vi "BRig_RT__Case_Exp__State_initBlock__v10.vi"(0 "input_dataCurrent":u16[](array[numeric]), 3 "input_dataExp":u16[](array[numeric]), 4 "input_dataBlock":u16[][](array[numeric]), 5 "input_dataTrial":u16[][](array[numeric])) -> (6 "output_iSpout":u16, 7 "output_speaker_amp_R":u16, 8 "output_iBlock":u16, 9 "output_speaker_freq_R":u8, 10 "output_BUR_target":u16, 11 "output_speaker_amp_L":u16, 12 "output_TpB_target":u16, 13 "output_speaker_freq_L":u8, 14 "output_dataCurrent":u16[](array[numeric]), 18 "output_dataBlock":u16[][](array[numeric]), 19 "output_dataTrial":u16[][](array[numeric]))   [LabVIEW 2014]
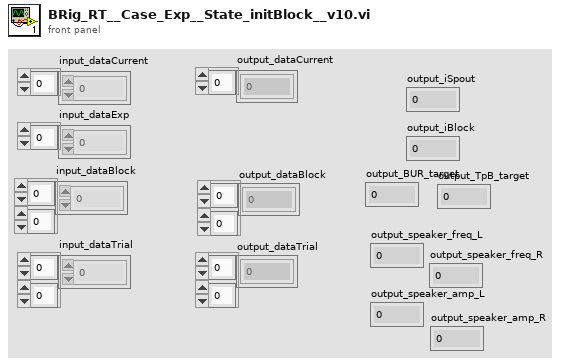
[diagram p1: front panel]
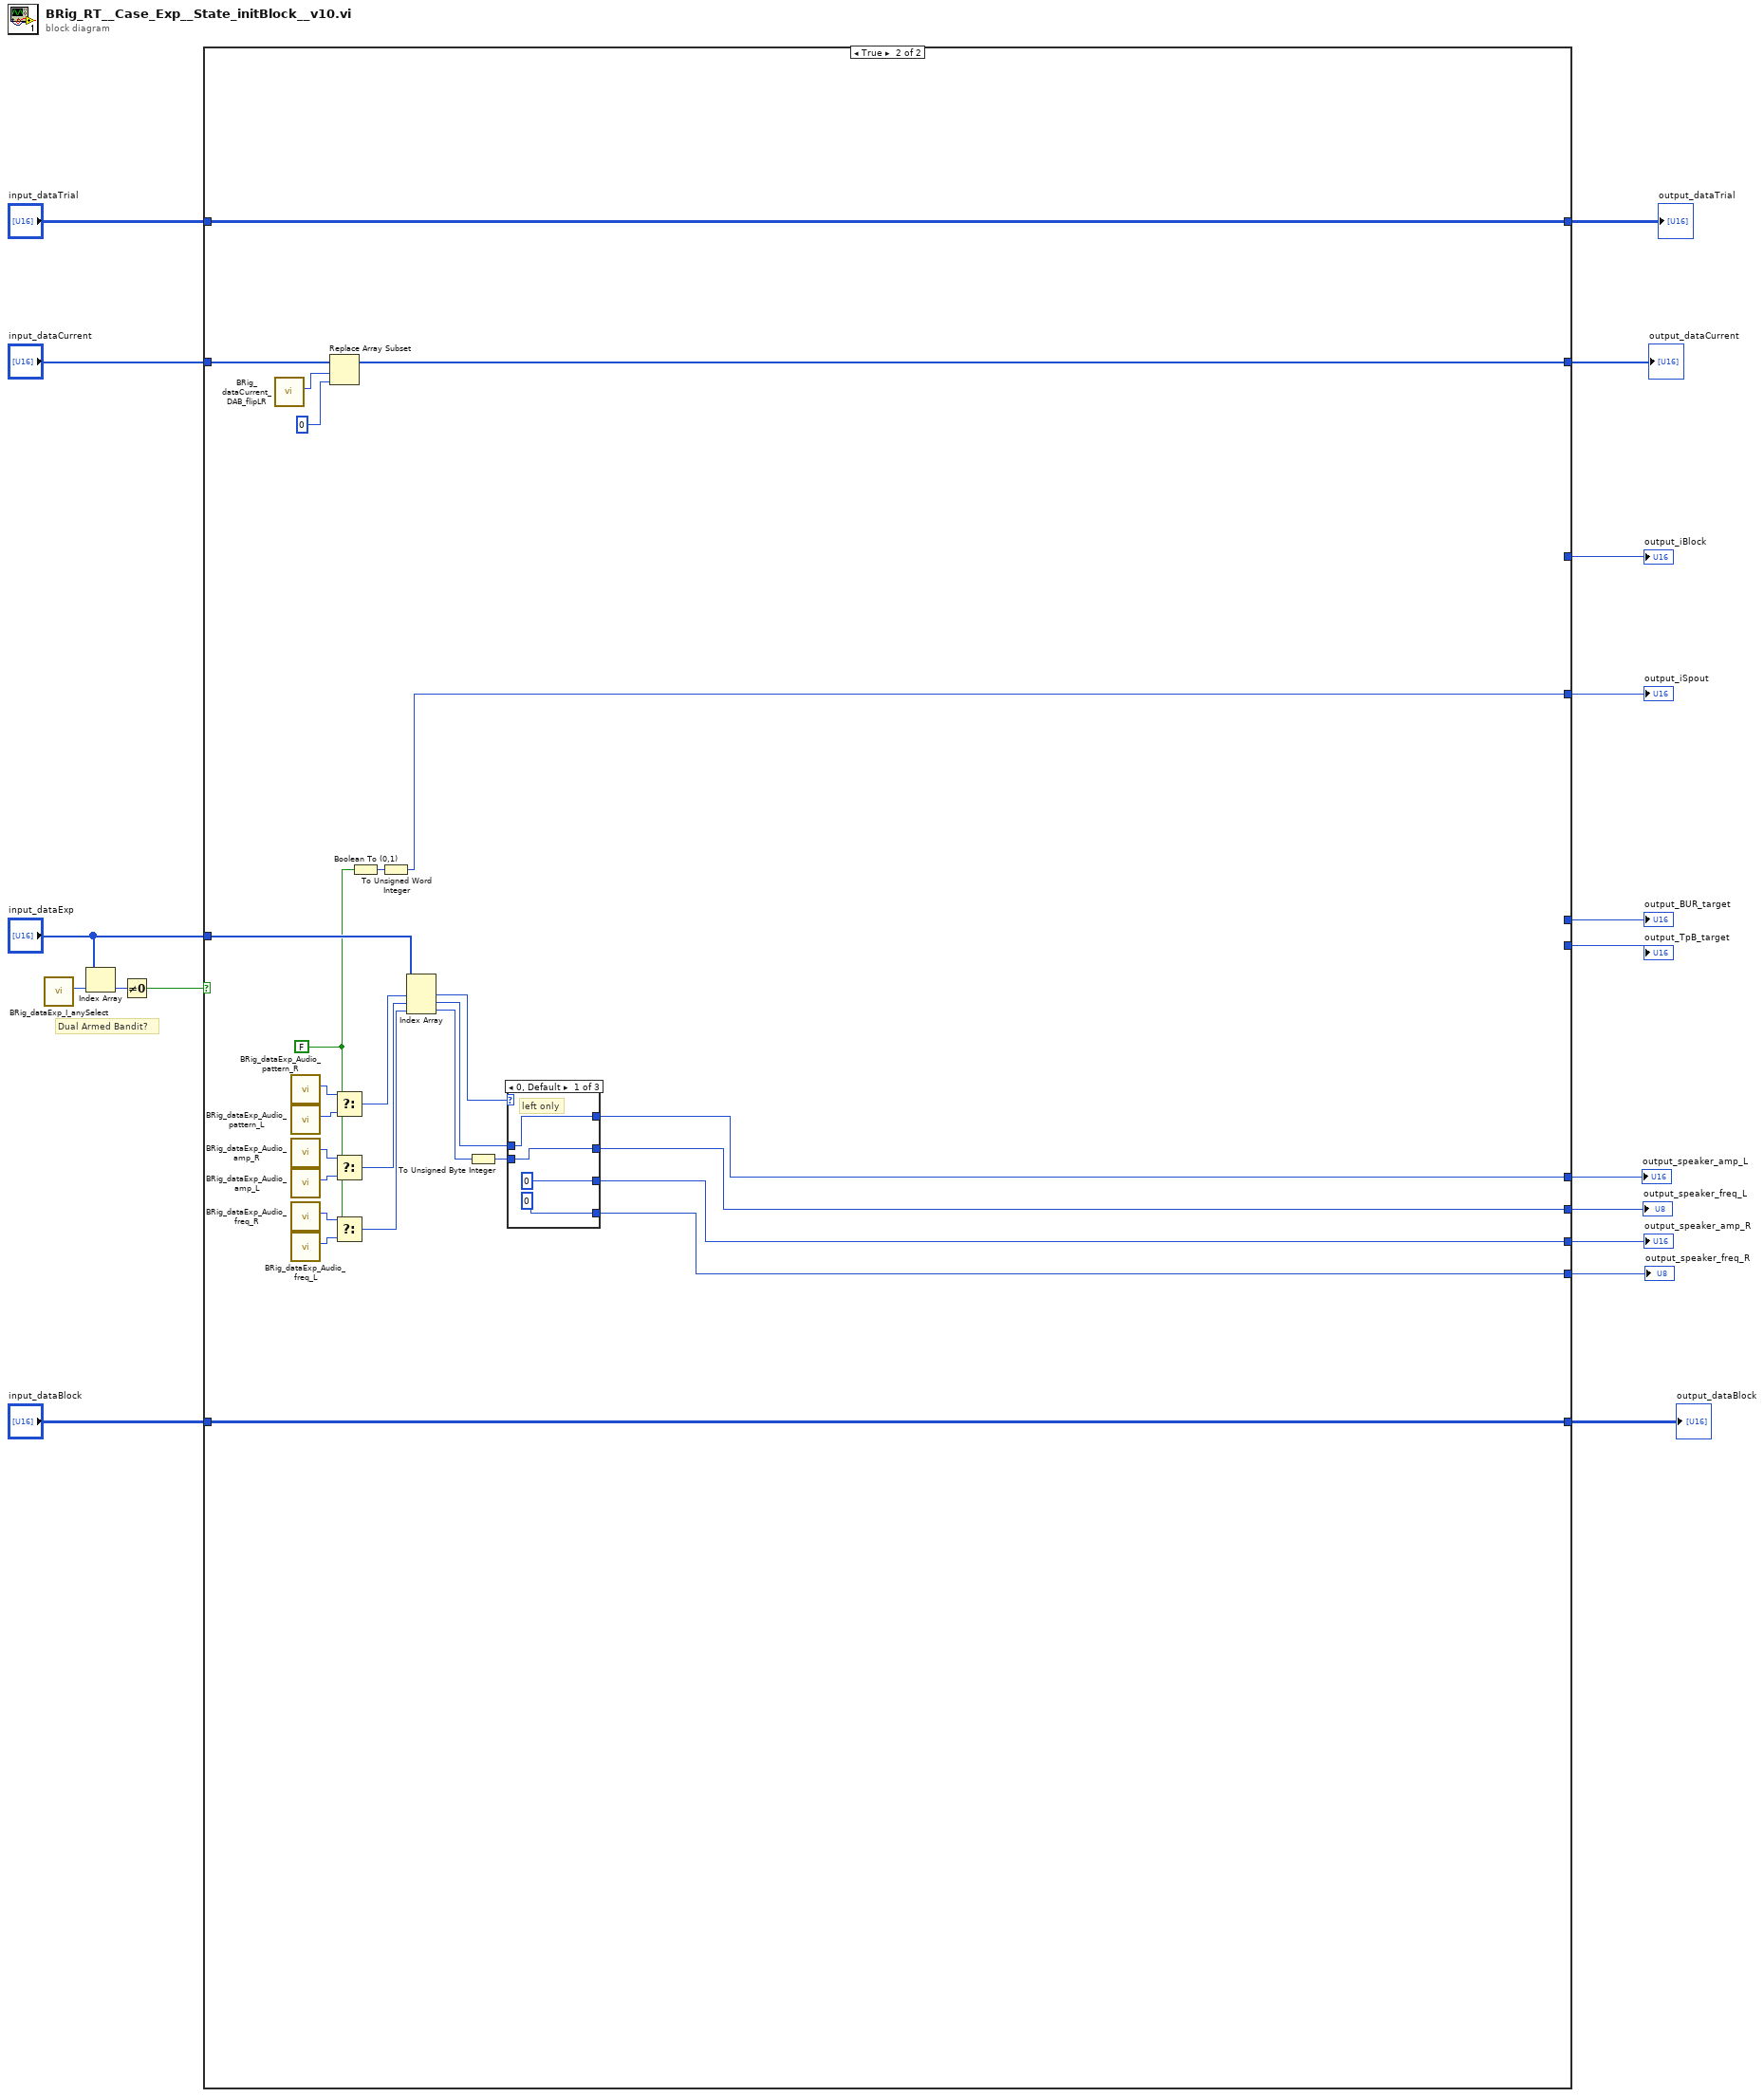
[diagram p0: block diagram]
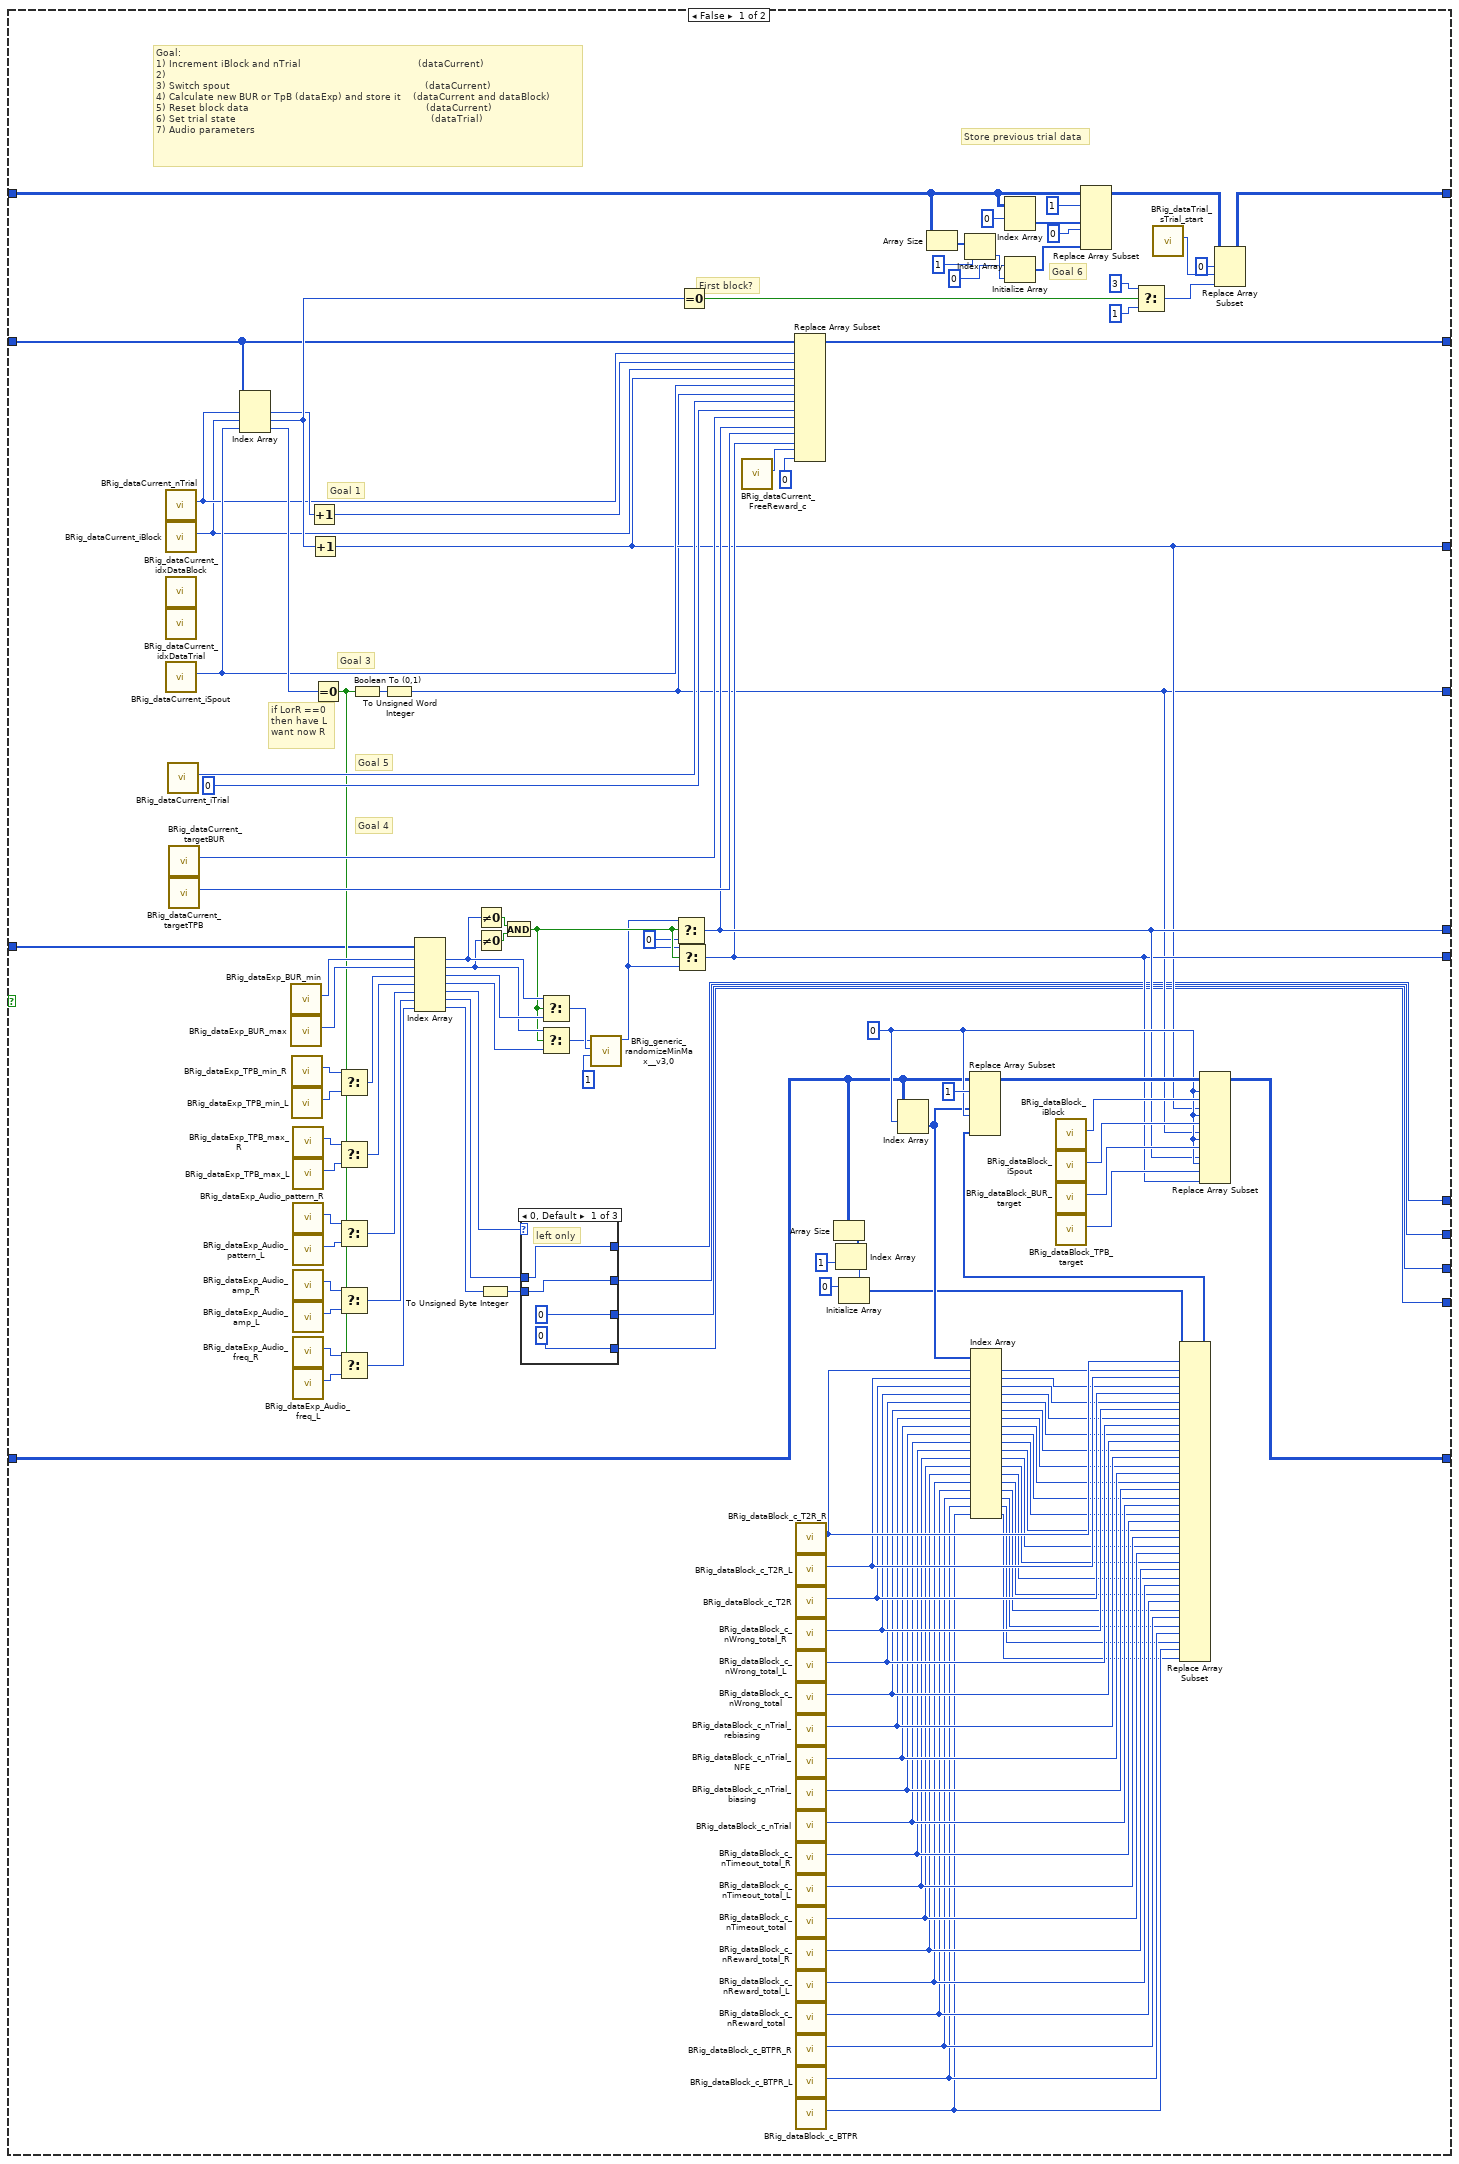
[diagram p2: hidden frame]
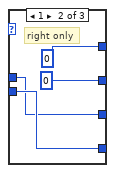
[diagram p3: hidden frame]
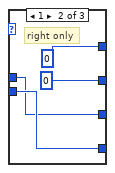
[diagram p5: hidden frame]
diagram:
  # "Dual Armed Bandit?"
  n1 = call "BRig_dataExp_I_anySelect.vi"() -> ("output_I_anySelect"=w17:i32)  [unwired: 11 in]
  n2 = Index Array(array="input_dataExp", index=w17) -> (element=w16:u16)
  n3 = Not Equal To 0?(x=w16) -> (x != 0?=w15:bool)
  n4 = case shown="True" w15 {
    tunnel: "input_dataExp" -> [w33 w171]
    tunnel: [w32 _] -> w14
    tunnel: [w31 _] -> w13
    tunnel: [w30 _] -> w12
    tunnel: [w29 w164] -> w11
    tunnel: "input_dataBlock" -> [w28 w186]
    tunnel: [w27 w186] -> w9
    tunnel: "input_dataTrial" -> [w26 w185]
    tunnel: "input_dataCurrent" -> [w25 w163]
    tunnel: [w24 w185] -> w6
    tunnel: [w23 w162] -> w5
    tunnel: [w22 w170] -> w4
    tunnel: [w21 w169] -> w3
    tunnel: [w20 w168] -> w2
    tunnel: [w19 w167] -> w1
    frame False {
      w75 = 0 ("disabled index (row)")
      w131 = u16 0 ("f")
      # "Store previous trial data"
      # "if LorR ==0\nthen have L\nwant now R"
      # "First block?"
      # "Goal 6"
      # "Goal 4"
      # "Goal 5"
      # "Goal 3"
      # "Goal 1"
      # "Goal:\n1) Increment iBlock and nTrial                                       (dataCurrent)\n2) \n3) Switch spout                                                                 (dataCurrent)\n4) Calculate new BUR or TpB (dataExp) and store it    (dataCurrent and dataBlock)\n5) Reset block data                                                           (dataCurrent)\n6) Set trial state                                                                 (dataTrial)\n7) Audio parameters"
      n5 = call "BRig_dataCurrent_nTrial.vi"() -> ("output_nTrial"=w94:i32)  [unwired: 11 in]
      n6 = call "BRig_dataCurrent_iBlock.vi"() -> ("output_iBlock"=w92:i32)  [unwired: 11 in]
      n7 = call "BRig_dataCurrent_idxDataBlock.vi"() -> ()  [unwired: 11 in, 1 out]
      n8 = call "BRig_dataCurrent_idxDataTrial.vi"() -> ()  [unwired: 11 in, 1 out]
      n9 = call "BRig_dataCurrent_iSpout.vi"() -> ("output_iSpout"=w116:i32)  [unwired: 11 in]
      n10 = call "BRig_dataCurrent_iTrial.vi"() -> ("output_iTrial"=w117:i32)  [unwired: 11 in]
      n11 = call "BRig_dataCurrent_targetBUR.vi"() -> ("output_targetBUR"=w119:i32)  [unwired: 11 in]
      n12 = call "BRig_dataCurrent_targetTPB.vi"() -> ("output_targetTPB"=w120:i32)  [unwired: 11 in]
      n13 = Index Array(array=w25, index #1=w94, index #2=w92, index #3=w116) -> (element #1=w115:u16, element #2=w125:u16, element #3=w148:u16)
      n14 = call "BRig_dataExp_BUR_min.vi"() -> ("output_BUR_min"=w147:i32)  [unwired: 11 in]
      n15 = call "BRig_dataExp_BUR_max.vi"() -> ("output_BUR_max"=w146:i32)  [unwired: 11 in]
      n16 = call "BRig_dataExp_TPB_min_R.vi"() -> ("output_TPB_min_R"=w143:i32)  [unwired: 11 in]
      n17 = call "BRig_dataExp_TPB_min_L.vi"() -> ("output_TPB_min_L"=w142:i32)  [unwired: 11 in]
      n18 = call "BRig_dataExp_TPB_max_R.vi"() -> ("output_TPB_max_R"=w97:i32)  [unwired: 11 in]
      n19 = call "BRig_dataExp_TPB_max_L.vi"() -> ("output_TPB_max_L"=w96:i32)  [unwired: 11 in]
      n20 = call "BRig_dataExp_Audio_pattern_R.vi"() -> ("output_Audio_sp__R"=w113:i32)  [unwired: 11 in]
      n21 = call "BRig_dataExp_Audio_pattern_L.vi"() -> ("output_Audio_sp__L"=w112:i32)  [unwired: 11 in]
      n22 = call "BRig_dataExp_Audio_amp_R.vi"() -> ("output_Audio_amp__R"=w111:i32)  [unwired: 11 in]
      n23 = call "BRig_dataExp_Audio_amp_L.vi"() -> ("output_Audio_amp__L"=w110:i32)  [unwired: 11 in]
      n24 = call "BRig_dataExp_Audio_freq_R.vi"() -> ("output_Audio_freq__R"=w109:i32)  [unwired: 11 in]
      n25 = call "BRig_dataExp_Audio_freq_L.vi"() -> ("output_Audio_freq__L"=w108:i32)  [unwired: 11 in]
      n26 = Increment(x=w115) -> (x+1=w93:u16)
      n27 = Increment(x=w125) -> (x+1=w30:u16)
      n28 = Equal To 0?(x=w148) -> (x = 0?=w114:bool)
      n29 = Select(t=w143, s=w114, f=w142) -> (s? t:f=w141:i32)
      n30 = Select(t=w97, s=w114, f=w96) -> (s? t:f=w140:i32)
      n31 = Select(t=w113, s=w114, f=w112) -> (s? t:f=w107:i32)
      n32 = Select(t=w111, s=w114, f=w110) -> (s? t:f=w106:i32)
      n33 = Select(t=w109, s=w114, f=w108) -> (s? t:f=w105:i32)
      n34 = Boolean To (0,1)(Boolean=w114) -> (0, 1=w149:i16)
      n35 = To Unsigned Word Integer(number=w149) -> (unsigned 16bit integer=w29:u16)
      n36 = Index Array(array=w33, index #1=w147, index #2=w146, index #3=w141, index #4=w140, index #5=w107, index #6=w106, index #7=w105) -> (element #1=w139:u16, element #2=w137:u16, element #3=w138:u16, element #4=w136:u16, element #5=w104:u16, element #6=w103:u16, element #7=w102:u16)
      n37 = Not Equal To 0?(x=w139) -> (x != 0?=w144:bool)
      n38 = Not Equal To 0?(x=w137) -> (x != 0?=w145:bool)
      n39 = To Unsigned Byte Integer(number=w102) -> (unsigned 8bit integer=w101:u8)
      n40 = And(x=w144, y=w145) -> (x .and. y?=w132:bool)
      n41 = case shown="0, Default" w104 {
        tunnel: w103 -> [w153 w156 w158]
        tunnel: w101 -> [w152 w157 w159]
        tunnel: [w153 u16 0 ("Numeric") w158] -> w22
        tunnel: [w152 u8 0 w159] -> w21
        tunnel: [u8 0 w157 w159] -> w19
        tunnel: [u16 0 ("Numeric") w156 w158] -> w20
        frame 0, Default {
          # "left only"
        }
        frame 1 {
          # "right only"
        }
        frame 2 {
          # "left and right"
        }
      }
      n42 = Select(t=w139, s=w132, f=w138) -> (s? t:f=w134:u16)
      n43 = Select(t=w137, s=w132, f=w136) -> (s? t:f=w133:u16)
      n44 = call "BRig_generic_randomizeMinMax__v3,0.vi"("Input_Increment"=u16 1, "Input_Min"=w134, "Input_Max"=w133) -> ("Output"=w130:u16)  [unwired: 8 in]
      n45 = Select(t=w130, s=w132, f=w131) -> (s? t:f=w32:u16)
      n46 = Select(t=w131, s=w132, f=w130) -> (s? t:f=w31:u16)
      n47 = Equal To 0?(x=w125) -> (x = 0?=w100:bool)
      n48 = call "BRig_dataCurrent_FreeReward_c.vi"() -> ("output_FreeReward_c"=w99:i32)  [unwired: 11 in]
      n49 = Replace Array Subset(array=w25, new element #1=w93, index #1=w94, new element #2=w30, index #2=w92, new element #3=w29, index #3=w116, new element #4=u16 0 ("new element/subarray"), index #4=w117, new element #5=w32, index #5=w119, new element #6=w31, index #6=w120, new element #7=u16 0 ("new element/subarray"), index #7=w99) -> (w23:u16[])
      n50 = call "BRig_dataBlock_c_T2R_R.vi"() -> ("output_c_T2R_R"=w71:i32)  [unwired: 11 in]
      n51 = call "BRig_dataBlock_c_T2R_L.vi"() -> ("output_c_T2R_L"=w70:i32)  [unwired: 11 in]
      n52 = call "BRig_dataBlock_c_T2R.vi"() -> ("output_c_T2R"=w69:i32)  [unwired: 11 in]
      n53 = call "BRig_dataBlock_c_nWrong_total_R.vi"() -> ("output_c_nWrong_total_R"=w68:i32)  [unwired: 11 in]
      n54 = call "BRig_dataBlock_c_nWrong_total_L.vi"() -> ("output_c_nWrong_total_L"=w67:i32)  [unwired: 11 in]
      n55 = call "BRig_dataBlock_c_nWrong_total.vi"() -> ("output_c_nWrong_total"=w66:i32)  [unwired: 11 in]
      n56 = call "BRig_dataBlock_c_nTrial_rebiasing.vi"() -> ("output_c_nTrial_rebiasing"=w65:i32)  [unwired: 11 in]
      n57 = call "BRig_dataBlock_c_nTrial_NFE.vi"() -> ("output_c_nTrial_NFE"=w64:i32)  [unwired: 11 in]
      n58 = call "BRig_dataBlock_c_nTrial_biasing.vi"() -> ("output_c_nTrial_biasing"=w63:i32)  [unwired: 11 in]
      n59 = call "BRig_dataBlock_c_nTrial.vi"() -> ("output_c_nTrial"=w62:i32)  [unwired: 11 in]
      n60 = call "BRig_dataBlock_c_nTimeout_total_R.vi"() -> ("output_c_nTimeout_total_R"=w61:i32)  [unwired: 11 in]
      n61 = call "BRig_dataBlock_c_nTimeout_total_L.vi"() -> ("output_c_nTimeout_total_L"=w60:i32)  [unwired: 11 in]
      n62 = call "BRig_dataBlock_c_nTimeout_total.vi"() -> ("output_c_nTimeout_total"=w59:i32)  [unwired: 11 in]
      n63 = call "BRig_dataBlock_c_nReward_total_R.vi"() -> ("output_nReward_total_R"=w58:i32)  [unwired: 11 in]
      n64 = call "BRig_dataBlock_c_nReward_total_L.vi"() -> ("output_nReward_total_L"=w57:i32)  [unwired: 11 in]
      n65 = call "BRig_dataBlock_c_nReward_total.vi"() -> ("output_nReward_total"=w56:i32)  [unwired: 11 in]
      n66 = call "BRig_dataBlock_c_BTPR_R.vi"() -> ("output_c_BTPR_R"=w55:i32)  [unwired: 11 in]
      n67 = call "BRig_dataBlock_c_BTPR_L.vi"() -> ("output_c_BTPR_L"=w54:i32)  [unwired: 11 in]
      n68 = call "BRig_dataBlock_c_BTPR.vi"() -> ("output_c_BTPR"=w53:i32)  [unwired: 11 in]
      n69 = Array Size(array=w28) -> (size(s)=w81:i32[])
      n70 = Index Array(array=w81, index=1) -> (element=w79:i32)
      n71 = Initialize Array(u16 0 ("index"), w79) -> (w73:u16[])
      n72 = Index Array(array=w28, index (row)=w75) -> (element=w74:u16[])  [unwired: 1 in]
      n73 = Array Size(array=w26) -> (size(s)=w86:i32[])
      n74 = Index Array(array=w86, index=1) -> (element=w84:i32)
      n75 = Index Array(array=w74, index #1=w71, index #2=w70, index #3=w69, index #4=w68, index #5=w67, index #6=w66, index #7=w65, index #8=w64, index #9=w63, index #10=w62, index #11=w61, index #12=w60, index #13=w59, index #14=w58, index #15=w57, index #16=w56, index #17=w55, index #18=w54, index #19=w53) -> (element #1=w34:u16, element #2=w35:u16, element #3=w36:u16, element #4=w37:u16, element #5=w38:u16, element #6=w39:u16, element #7=w40:u16, element #8=w41:u16, element #9=w42:u16, element #10=w43:u16, element #11=w44:u16, element #12=w45:u16, element #13=w46:u16, element #14=w47:u16, element #15=w48:u16, element #16=w49:u16, element #17=w50:u16, element #18=w51:u16, element #19=w52:u16)
      n76 = Index Array(array=w26, index (row)=0) -> (element=w88:u16[])  [unwired: 1 in]
      n77 = Initialize Array(u16 0 ("index"), w84) -> (w82:u16[])
      n78 = call "BRig_dataBlock_iBlock.vi"() -> ("output_iBlock"=w129:i32)  [unwired: 11 in]
      n79 = call "BRig_dataBlock_iSpout.vi"() -> ("output_iSpout"=w128:i32)  [unwired: 11 in]
      n80 = call "BRig_dataBlock_BUR_target.vi"() -> ("output_BUR_target"=w127:i32)  [unwired: 11 in]
      n81 = call "BRig_dataBlock_TPB_target.vi"() -> ("output_TPB_target"=w126:i32)  [unwired: 11 in]
      n82 = Replace Array Subset(array=w26, new element #1=w88, index (row) #1=1 ("index (row)"), new element #2=w82, index (row) #2=0 ("index (row)")) -> (w91:u16[][])  [unwired: 2 in]
      n83 = Select(t=u16 3 ("new element/subarray"), s=w100, f=u16 1 ("new element/subarray")) -> (s? t:f=w123:u16)
      n84 = call "BRig_dataTrial_sTrial_start.vi"() -> ("output_sTrial_start"=w124:i32)  [unwired: 11 in]
      n85 = Replace Array Subset(array=w73, new element #1=w34, index #1=w71, new element #2=w35, index #2=w70, new element #3=w36, index #3=w69, new element #4=w37, index #4=w68, new element #5=w38, index #5=w67, new element #6=w39, index #6=w66, new element #7=w40, index #7=w65, new element #8=w41, index #8=w64, new element #9=w42, index #9=w63, new element #10=w43, index #10=w62, new element #11=w44, index #11=w61, new element #12=w45, index #12=w60, new element #13=w46, index #13=w59, new element #14=w47, index #14=w58, new element #15=w48, index #15=w57, new element #16=w49, index #16=w56, new element #17=w50, index #17=w55, new element #18=w51, index #18=w54, new element #19=w52, index #19=w53) -> (w72:u16[])
      n86 = Replace Array Subset(array=w28, new element #1=w74, index (row) #1=1 ("index (row)"), new element #2=w72, index (row) #2=w75) -> (w76:u16[][])  [unwired: 2 in]
      n87 = Replace Array Subset(array=w76, new element #1=w30, index (row) #1=w75, index (col) #1=w129, new element #2=w29, index (row) #2=w75, index (col) #2=w128, new element #3=w32, index (row) #3=w75, index (col) #3=w127, new element #4=w31, index (row) #4=w75, index (col) #4=w126) -> (w27:u16[][])
      n88 = Replace Array Subset(array=w91, new element=w123, index (row)=0 ("disabled index (row)"), index (col)=w124) -> (w24:u16[][])
    }
    frame True {
      w165 = FALSE
      n89 = call "BRig_dataCurrent_DAB_flipLR.vi"() -> ("output_DAB_flipLR"=w161:i32)  [unwired: 11 in]
      n90 = call "BRig_dataExp_Audio_pattern_R.vi"() -> ("output_Audio_sp__R"=w184:i32)  [unwired: 11 in]
      n91 = call "BRig_dataExp_Audio_pattern_L.vi"() -> ("output_Audio_sp__L"=w183:i32)  [unwired: 11 in]
      n92 = call "BRig_dataExp_Audio_amp_R.vi"() -> ("output_Audio_amp__R"=w182:i32)  [unwired: 11 in]
      n93 = call "BRig_dataExp_Audio_amp_L.vi"() -> ("output_Audio_amp__L"=w181:i32)  [unwired: 11 in]
      n94 = call "BRig_dataExp_Audio_freq_R.vi"() -> ("output_Audio_freq__R"=w180:i32)  [unwired: 11 in]
      n95 = call "BRig_dataExp_Audio_freq_L.vi"() -> ("output_Audio_freq__L"=w179:i32)  [unwired: 11 in]
      n96 = Replace Array Subset(array=w163, new element=u16 0 ("new element/subarray"), index=w161) -> (w162:u16[])
      n97 = Select(t=w184, s=w165, f=w183) -> (s? t:f=w178:i32)
      n98 = Select(t=w182, s=w165, f=w181) -> (s? t:f=w177:i32)
      n99 = Select(t=w180, s=w165, f=w179) -> (s? t:f=w176:i32)
      n100 = Boolean To (0,1)(Boolean=w165) -> (0, 1=w166:i16)
      n101 = To Unsigned Word Integer(number=w166) -> (unsigned 16bit integer=w164:u16)
      n102 = Index Array(array=w171, index #1=w178, index #2=w177, index #3=w176) -> (element #1=w175:u16, element #2=w174:u16, element #3=w173:u16)
      n103 = To Unsigned Byte Integer(number=w173) -> (unsigned 8bit integer=w172:u8)
      n104 = case shown="0, Default" w175 {
        tunnel: w174 -> [w190 w193 w195]
        tunnel: w172 -> [w189 w194 w196]
        tunnel: [w190 u16 0 ("Numeric") w195] -> w170
        tunnel: [w189 u8 0 w196] -> w169
        tunnel: [u8 0 w194 w196] -> w167
        tunnel: [u16 0 ("Numeric") w193 w195] -> w168
        frame 0, Default {
          # "left only"
        }
        frame 1 {
          # "right only"
        }
        frame 2 {
          # "left and right"
        }
      }
    }
  }
  "output_BUR_target" <- w14
  "output_TpB_target" <- w13
  "output_iBlock" <- w12
  "output_iSpout" <- w11
  "output_dataBlock" <- w9
  "output_dataTrial" <- w6
  "output_dataCurrent" <- w5
  "output_speaker_amp_L" <- w4
  "output_speaker_freq_L" <- w3
  "output_speaker_amp_R" <- w2
  "output_speaker_freq_R" <- w1
